vi "Destroy.vi"(8 "error in (no error)":errorcluster, 11 "Writer (Greyscale) in":refnum<class "Writer (Greyscale).lvclass">) -> (0 "error out":errorcluster, 3 "Path":path)   [LabVIEW 2020, in "video_io.lvlib" / "Writer (Greyscale).lvclass"]
uses:
  Writer (Greyscale).lvclass
  Writer (Greyscale).lvclass/Writer (Greyscale).ctl
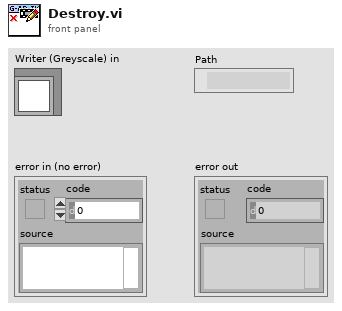
[diagram p1: front panel]
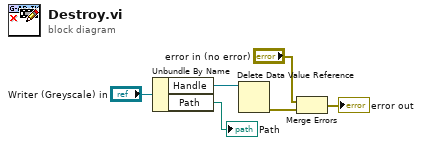
[diagram p0: block diagram]
diagram:
  n1 = Unbundle By Name("Writer (Greyscale) in") -> ("Handle"=w4:refnum<data-value>, "Path"=→"Path":path)
  n2 = Delete Data Value Reference(data value reference=w4) -> (error out=w2:errorcluster)  [unwired: 1 in, 1 out]
  n3 = Merge Errors("error in (no error)", w2) -> (→"error out":errorcluster)
